vi "PH_Interaction.Save String Data to Harddisk.vi"(0 "i ref in":refnum<vi>, 1 "Explanation (for Example: Column 1: xxx, ...)":string, 2 "Data (for example: Columns)":string, 3 "file name extension":T1="*.dat", 4 "start path (O:\\)":path=path "O:/", 5 "error in (no error)":errorcluster) -> (14 "i ref out":refnum<vi>, 17 "File Path":path, 19 "error out":errorcluster)   [LabVIEW 2014, in "PH_Common.lvlib"]
doc: "This VI writes data to the harddisk; stored data have a headline which instance saved the data (if the reference is valid) at which time. At explanation it can be explained what the data are; Data shall be strings. The file name extinction can also be selected, while the path is chosen interactively."
uses:
  PH_Common.lvlib
  Names/PH_Names.File Types.ctl
  CSCore/CSSystem/CSSystemLib/CSSystemLib.lvlib
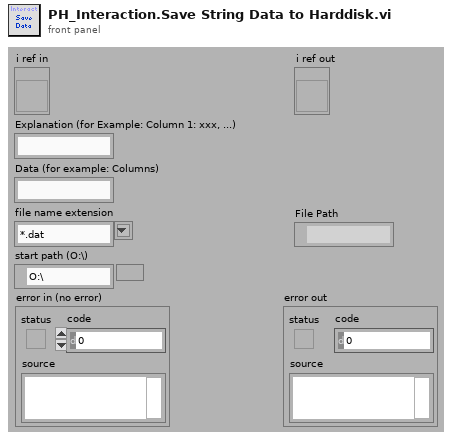
[diagram p1: front panel]
types:
  T1 = typedef "PH_Common.lvlib/PH_Names.File Types.ctl" = string
  T2 = enum16{"open", "replace", "create", "open or create", "replace or create", "replace or create with confirmation"}
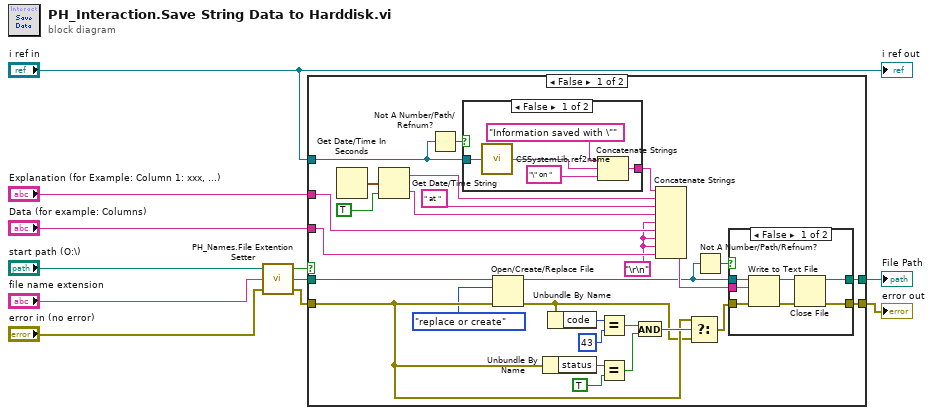
[diagram p0: block diagram]
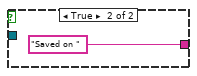
[diagram p2: hidden frame]
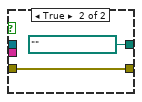
[diagram p3: hidden frame]
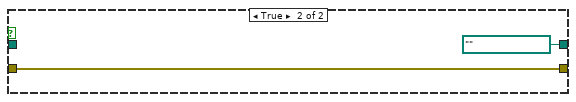
[diagram p4: hidden frame]
diagram:
  n1 = call "PH_Names.File Extention Setter.vi"("error in (no error)"="error in (no error)", "File Type"="file name extension", "start path (O:\\)"="start path (O:\\)") -> ("error out"=w2:errorcluster, "path with extension"=w8:path, "cancelled?"=w5:bool)
  n2 = case shown="False" w5 {
    tunnel: "Data (for example: Columns)" -> [w39 _]
    tunnel: "Explanation (for Example: Column 1: xxx, ...)" -> [w38 _]
    tunnel: w8 -> [w32 _]
    tunnel: [w31 w56] -> w7
    tunnel: w2 -> [w19 w56]
    tunnel: "i ref in" -> [w14 _]
    tunnel: [w12 path "" ("path")] -> w1
    frame False {
      w29 = "\r\n"
      n3 = Get Date/Time In Seconds() -> (seconds since 1Jan1904=w35:timestamp)
      n4 = Get Date/Time String(seconds (now)=w35, want seconds? (F)=TRUE) -> (date string=w36:string, time string=w37:string)  [unwired: 1 in]
      n5 = Not A Number/Path/Refnum?(number/path/refnum=w14) -> (NaN/Path/Refnum?=w15:bool)
      n6 = case shown="False" w15 {
        tunnel: w14 -> [w44 _]
        tunnel: [w40 "Saved on "] -> w16
        frame False {
          n7 = call "CSSystemLib.ref2name.vi"("obj refnum"=w44) -> ("name"=w42:string)
          n8 = Concatenate Strings("Information saved with \"" ("string"), w42, "\" on " ("string")) -> (w40:string)
        }
        frame True {
        }
      }
      n9 = Open/Create/Replace File(file path (use dialog)=w32, error in=w19, operation (0:open)=T2."replace or create") -> (refnum out=w27:refnum<file>, error out=w18:errorcluster)  [unwired: 3 in, 1 out]
      n10 = Unbundle By Name(w19) -> ("status"=w24:bool)
      n11 = Unbundle By Name(w18) -> ("code"=w26:i32)
      n12 = Equal?(x=w26, y=43) -> (x = y?=w22:bool)
      n13 = Equal?(x=w24, y=TRUE) -> (x = y?=w21:bool)
      n14 = And(x=w22, y=w21) -> (x .and. y?=w20:bool)
      n15 = Concatenate Strings(w16, w36, " at " ("string"), w37, w29, w38, w29, w29, w39) -> (w33:string)
      n16 = Select(t=w19, s=w20, f=w18) -> (s? t:f=w17:errorcluster)
      n17 = Not A Number/Path/Refnum?(number/path/refnum=w27) -> (NaN/Path/Refnum?=w28:bool)
      n18 = case shown="False" w28 {
        tunnel: w33 -> [w52 _]
        tunnel: w17 -> [w50 w54]
        tunnel: w27 -> [w48 _]
        tunnel: [w47 w54] -> w31
        tunnel: [w46 path "" ("path")] -> w12
        frame False {
          n19 = Write to Text File(file (use dialog)=w48, text=w52, error in=w50) -> (refnum out=w51:refnum<file>, error out=w49:errorcluster)  [unwired: 1 in, 1 out]
          n20 = Close File(refnum=w51, error in=w49) -> (path=w46:path, error out=w47:errorcluster)
        }
        frame True {
        }
      }
    }
    frame True {
    }
  }
  "error out" <- w7
  "File Path" <- w1
  "i ref out" <- "i ref in"
